vi "Day4Part2.vi"(11 "Input":string="MMMSXXMASM\nMSAMXMSMSA\nAMXSXMAAMM\nMSAMASMSMX\nXMASAMXAMM\nXXAMMXXAMA\nSMSMSASXSS\nSAXAMASAAA\nMAMMMXMMMM\nMXMXAXMASX") -> (3 "Result":i64)   [LabVIEW 2024]
uses:
  <userlib>/_OpenG.lib/string/string.llb/openg_string.lvlib
panel:
  out "Array":i64[][](array[numeric])
  out "Character Array":string[][](array[string])
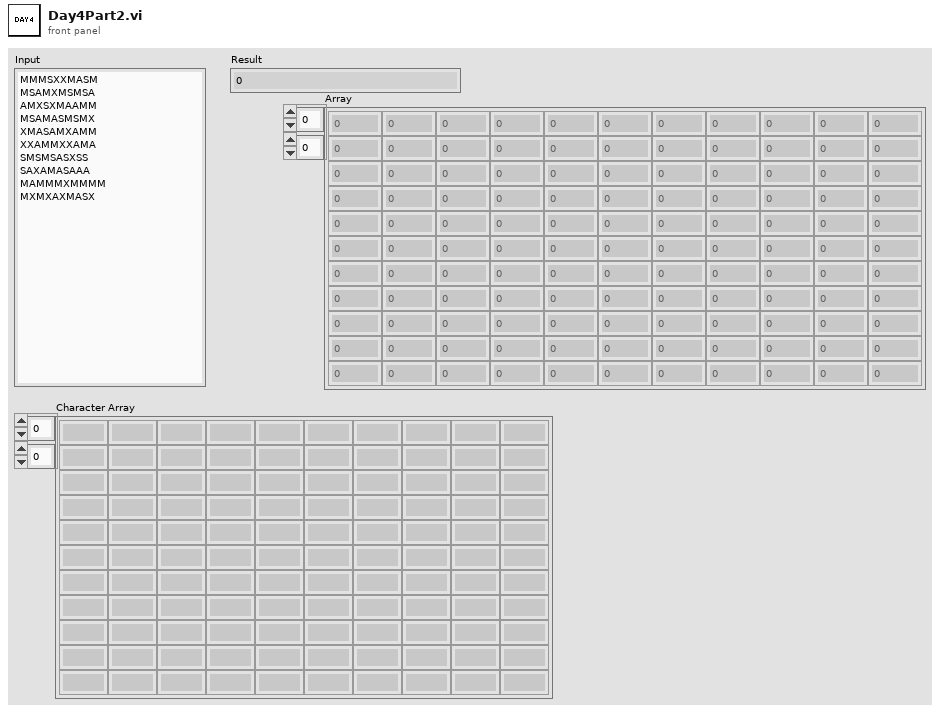
[diagram p1: front panel]
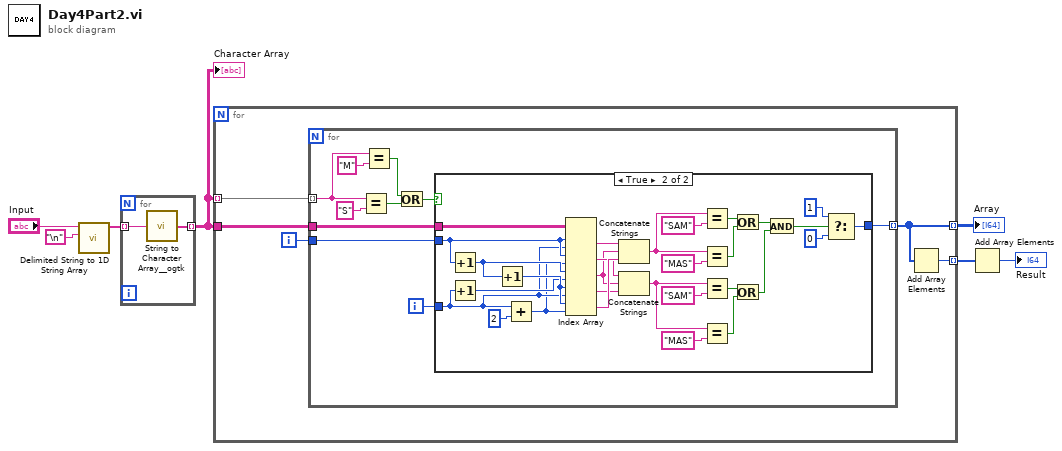
[diagram p0: block diagram]
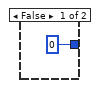
[diagram p2: hidden frame]
diagram:
  n1 = call <vilib>:"Delimited String to 1D String Array.vi"("delimiter"="\n", "delimited string"="Input") -> ("string array"=w5:string[])  [unwired: 9 in]
  n2 = for {
    tunnel: w5 -> [w9] mode=indexing
    tunnel: [w8] -> w2 mode=indexing
    n3 = call <userlib>:"String to Character Array__ogtk.vi"("Input String"=w9) -> ("Character Array"=w8:string[])
  }
  "Character Array" <- w2
  n4 = for {
    tunnel: w2 -> [w11] mode=indexing
    tunnel: w2 -> [w13]
    tunnel: [w12] -> w4 mode=indexing
    tunnel: [w10] -> w1 mode=indexing
    i -> [w14]
    n5 = for {
      tunnel: w14 -> [w21]
      tunnel: w13 -> [w24]
      tunnel: w11 -> [w17] mode=indexing
      tunnel: [w22] -> w10 mode=indexing
      i -> [w20]
      n6 = Equal?(x=w17, y="S") -> (x = y?=w16:bool)
      n7 = Equal?(x=w17, y="M") -> (x = y?=w19:bool)
      n8 = Or(x=w19, y=w16) -> (x .or. y?=w15:bool)
      n9 = case shown="True" w15 {
        tunnel: w24 -> [_ w54]
        tunnel: [0 w44] -> w22
        tunnel: w21 -> [_ w53]
        tunnel: w20 -> [_ w48]
        frame False {
        }
        frame True {
          n10 = Increment(x=w53) -> (x+1=w52:i32)
          n11 = Increment(x=w48) -> (x+1=w49:i32)
          n12 = Increment(x=w52) -> (x+1=w51:i32)
          n13 = Add(x=w48, y=2) -> (x+y=w47:i32)
          n14 = Index Array(array=w54, index (row) #1=w53, index (col) #1=w48, index (row) #2=w53, index (col) #2=w47, index (row) #3=w52, index (col) #3=w49, index (row) #4=w51, index (col) #4=w48, index (row) #5=w51, index (col) #5=w47) -> (element #1=w32:string, element #2=w29:string, element #3=w28:string, element #4=w27:string, element #5=w31:string)
          n15 = Concatenate Strings(w32, w28, w31) -> (w30:string)
          n16 = Concatenate Strings(w29, w28, w27) -> (w26:string)
          n17 = Equal?(x=w30, y="SAM") -> (x = y?=w35:bool)
          n18 = Equal?(x=w30, y="MAS") -> (x = y?=w34:bool)
          n19 = Equal?(x=w26, y="SAM") -> (x = y?=w41:bool)
          n20 = Equal?(x=w26, y="MAS") -> (x = y?=w40:bool)
          n21 = Or(x=w35, y=w34) -> (x .or. y?=w33:bool)
          n22 = Or(x=w41, y=w40) -> (x .or. y?=w39:bool)
          n23 = And(x=w33, y=w39) -> (x .and. y?=w38:bool)
          n24 = Select(t=1, s=w38, f=0) -> (s? t:f=w44:i32)
        }
      }
    }
    n25 = Add Array Elements(numeric array=w10) -> (sum=w12:i32)
  }
  "Array" <- w1
  n26 = Add Array Elements(numeric array=w4) -> (sum=→"Result":i32)
